vi "steptest-sorensen.vi"() -> ()   [LabVIEW 2017]
panel:
  out "3bit":bool
  out "2bit":bool
  out "1bit":bool
  out "0bit":bool
  in  "Direction":bool
  out "Count":i32
  out "Boolean array":bool[](array[boolean])
  in  "stop":bool
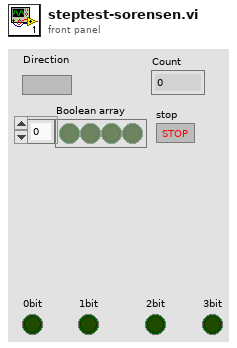
[diagram p1: front panel]
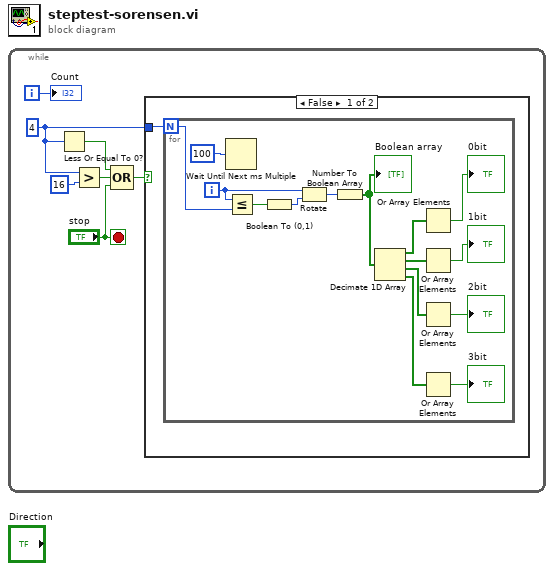
[diagram p0: block diagram]
diagram:
  n1 = while {
    i -> [w7]
    stop <- "stop" stop-if-true
    w2 = 4 ("Number of btis")
    n2 = Less Or Equal To 0?(x=w2) -> (x <= 0?=w6:bool)
    n3 = Greater?(x=w2, y=16) -> (0:w5:bool)
    n4 = Compound Arithmetic op=OR(w6, w5, "stop") -> (w4:bool)
    n5 = case shown="False" w4 {
      tunnel: w2 -> [w8 _]
      frame False {
        n6 = for {
          N: w8 -> [w18]
          i -> [w20]
          n7 = Wait Until Next ms Multiple(millisecond multiple=u32 100) -> ()  [unwired: 1 out]
          n8 = Less Or Equal?(x=w20, y=w18) -> (x <= y?=w22:bool)
          n9 = Boolean To (0,1)(Boolean=w22) -> (0, 1=w21:i16)
          n10 = Rotate(1:w21, 2:w20) -> (0:w23:i16)
          n11 = Number To Boolean Array(number=w23) -> (Boolean array=w17:bool[])
          "Boolean array" <- w17
          n12 = Decimate 1D Array(w17) -> (w16:bool[], w14:bool[], w13:bool[], w12:bool[])
          n13 = Or Array Elements(Boolean array=w16) -> (logical OR=→"0bit":bool)
          n14 = Or Array Elements(Boolean array=w14) -> (logical OR=→"1bit":bool)
          n15 = Or Array Elements(Boolean array=w13) -> (logical OR=→"2bit":bool)
          n16 = Or Array Elements(Boolean array=w12) -> (logical OR=→"3bit":bool)
        }
      }
      frame True {
      }
    }
    "Count" <- w7
  }
